vi "Run Bfr Tx - FIFO Payload.vi"(6 "Data in":u8[](array[numeric]), 8 "error in (no error)":errorcluster, 9 "Data Size":i32, 11 "Offset in":u64) -> (0 "error out":errorcluster, 3 "Offset out":u64, 4 "Data out":u8[](array[numeric]))   [LabVIEW 2019, in "UDP-Custom-Device Engine.lvlib"]
uses:
  UDP-Custom-Device Engine.lvlib
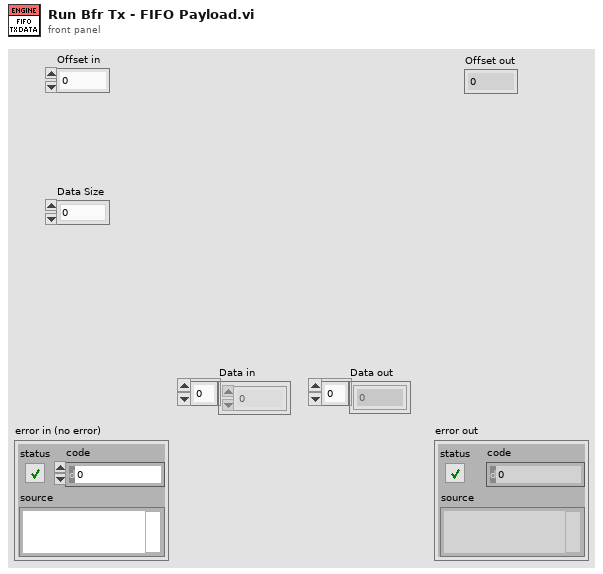
[diagram p1: front panel]
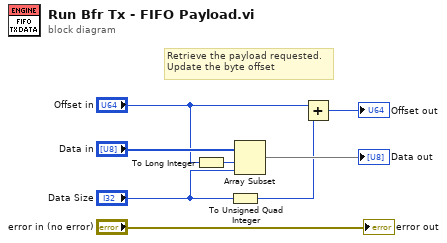
[diagram p0: block diagram]
diagram:
  # "Retrieve the payload requested.\nUpdate the byte offset"
  n1 = To Long Integer(number="Offset in") -> (32bit integer=w6:i32)
  n2 = To Unsigned Quad Integer(1:"Data Size") -> (0:w2:u64)
  n3 = Array Subset(array="Data in", index=w6, length="Data Size") -> (→"Data out":u8[])
  n4 = Add(x="Offset in", y=w2) -> (x+y=→"Offset out":u64)
  "error out" <- "error in (no error)"
